vi "Search Content For Database.vi"(8 "error in (no error)":errorcluster, 11 "searchContent":T1) -> (0 "error out":errorcluster, 3 "Query":string)   [LabVIEW 2015, in "UserManagement.lvlib" / "UserBasicInfo.lvclass"]
doc: "Functions : <b> Member search built in this vi!"
uses:
  UserManagement/UserBasicInfo/UserBasicInfo.lvclass
  typedef/Member Search Condition(UI).ctl
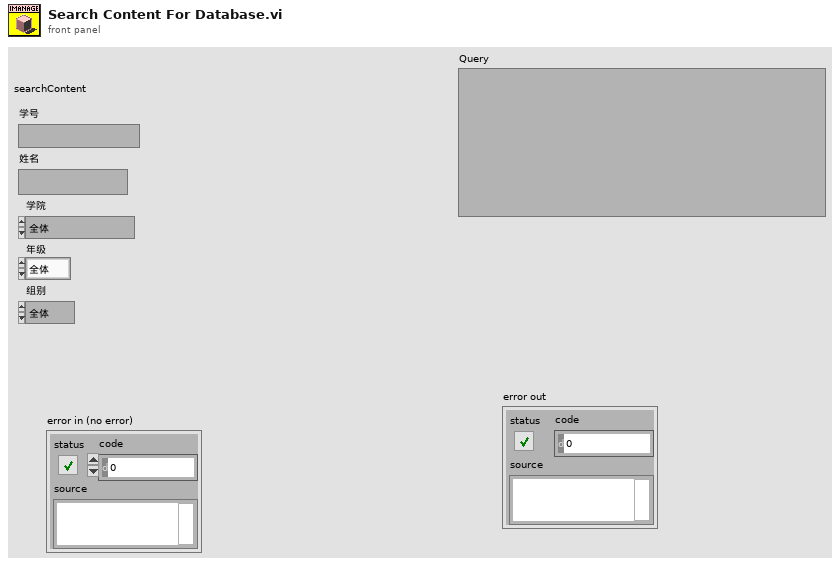
[diagram p1: front panel]
types:
  T1 = typedef "UserManagement.lvlib/UserBasicInfo.lvclass/Member Search Condition(UI).ctl" = cluster{"学号":string, "姓名":string, "学院":enum16{"全体", "机电工程学院", "电气工程学院", "航天学院", "能源学院", "理学院", "英才学院"}, "年级":enum16{"全体", "大二", "大三", "大四", "研一"}, "组别":enum16{"全体", "电控", "机械", "视觉"}}
  T2 = enum16{"全体", "机电工程学院", "电气工程学院", "航天学院", "能源学院", "理学院", "英才学院"}
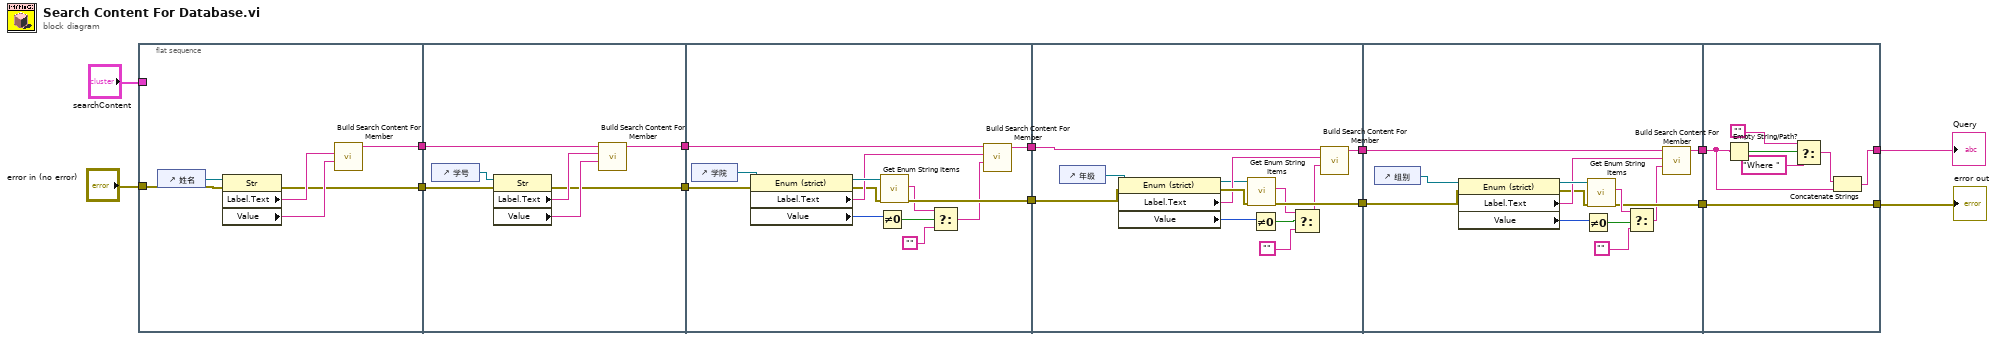
[diagram p0: block diagram]
diagram:
  n1 = flat-sequence {
    tunnel: [w20] -> w13
    tunnel: "searchContent" -> [_]
    tunnel: [w16] -> w11
    tunnel: "error in (no error)" -> [w15]
    tunnel: w13 -> [w27]
    tunnel: w11 -> [w26]
    tunnel: [w23] -> w10
    tunnel: [w22] -> w9
    tunnel: w10 -> [w37]
    tunnel: w9 -> [w40]
    tunnel: [w34] -> w8
    tunnel: [w33] -> w7
    tunnel: w8 -> [w49]
    tunnel: w7 -> [w48]
    tunnel: [w47] -> w6
    tunnel: [w46] -> w5
    tunnel: w6 -> [w62]
    tunnel: w5 -> [w61]
    tunnel: [w60] -> w2
    tunnel: [w56] -> w1
    tunnel: [w73] -> w4
    tunnel: [w67] -> w14
    tunnel: w2 -> [w68]
    tunnel: w1 -> [w73]
    frame #0 {
      n2 = control-ref of="姓名"() -> (w19:refnum<vi>)
      n3 = property class="Str"(reference=w19, error in=w15) -> (error out=w16:errorcluster, "Label.Text"=w18:string, "Value"=w17:string)  [unwired: 1 out]
      n4 = call "Build Search Content For Member.vi"("ItemContent"=w17, "ItemHeader"=w18) -> ("Result"=w20:string)  [unwired: 8 in]
    }
    frame #1 {
      n5 = control-ref of="学号"() -> (w21:refnum<vi>)
      n6 = property class="Str"(reference=w21, error in=w26) -> (error out=w23:errorcluster, "Label.Text"=w25:string, "Value"=w24:string)  [unwired: 1 out]
      n7 = call "Build Search Content For Member.vi"("ItemContent"=w24, "ItemHeader"=w25, "Source"=w27) -> ("Result"=w22:string)  [unwired: 7 in]
    }
    frame #2 {
      n8 = control-ref of="学院"() -> (w38:refnum<vi>)
      n9 = property class="Enum (strict)"(reference=w38, error in=w37) -> (reference out=w39:refnum<vi>, error out=w35:errorcluster, "Label.Text"=w36:string, "Value"=w32:T2)
      n10 = Not Equal To 0?(x=w32) -> (x != 0?=w31:bool)
      n11 = call "Get Enum String Items.vi"("error in (no error)"=w35, "Enum Refnum"=w39) -> ("error out"=w33:errorcluster, "String"=w30:string)  [unwired: 7 in]
      n12 = Select(t=w30, s=w31, f="") -> (s? t:f=w28:string)
      n13 = call "Build Search Content For Member.vi"("ItemContent"=w28, "ItemHeader"=w36, "Source"=w40) -> ("Result"=w34:string)  [unwired: 7 in]
    }
    frame #3 {
      n14 = control-ref of="年级"() -> (w51:refnum<vi>)
      n15 = property class="Enum (strict)"(reference=w51, error in=w48) -> (reference out=w50:refnum<vi>, error out=w53:errorcluster, "Label.Text"=w52:string, "Value"=w45:enum16{"全体", "大二", "大三", "大四", "研一"})
      n16 = call "Get Enum String Items.vi"("error in (no error)"=w53, "Enum Refnum"=w50) -> ("error out"=w47:errorcluster, "String"=w43:string)  [unwired: 7 in]
      n17 = Not Equal To 0?(x=w45) -> (x != 0?=w44:bool)
      n18 = Select(t=w43, s=w44, f="") -> (s? t:f=w41:string)
      n19 = call "Build Search Content For Member.vi"("ItemContent"=w41, "ItemHeader"=w52, "Source"=w49) -> ("Result"=w46:string)  [unwired: 7 in]
    }
    frame #4 {
      n20 = control-ref of="组别"() -> (w65:refnum<vi>)
      n21 = property class="Enum (strict)"(reference=w65, error in=w62) -> (reference out=w66:refnum<vi>, error out=w63:errorcluster, "Label.Text"=w64:string, "Value"=w59:enum16{"全体", "电控", "机械", "视觉"})
      n22 = Not Equal To 0?(x=w59) -> (x != 0?=w58:bool)
      n23 = call "Get Enum String Items.vi"("error in (no error)"=w63, "Enum Refnum"=w66) -> ("error out"=w56:errorcluster, "String"=w57:string)  [unwired: 7 in]
      n24 = Select(t=w57, s=w58, f="") -> (s? t:f=w54:string)
      n25 = call "Build Search Content For Member.vi"("ItemContent"=w54, "ItemHeader"=w64, "Source"=w61) -> ("Result"=w60:string)  [unwired: 7 in]
    }
    frame #5 {
      n26 = Empty String/Path?(string/path=w68) -> (empty?=w72:bool)
      n27 = Select(t="", s=w72, f="Where ") -> (s? t:f=w69:string)
      n28 = Concatenate Strings(w69, w68) -> (w67:string)
    }
  }
  "Query" <- w14
  "error out" <- w4
